vi "CRYCustom Curve Name Replace.vi"(8 "Hardware in":string, 9 "Step Setup in":string, 10 "Setup in":T1={"No.VI"=0, "Category"="", "StepName"="", "Seq setup flattened"="", "Comment"="", "Steps config."=[], "Jump config"=[], "Start"=0.0, "Increment"=0.0, "Name"="Pa", "Unit"="Pa", "Y data"=1, "Y prefix"="", "Y dB ref"=1.0, "Y unit"="", "Repeat State Array"=[]} {"Repeat State Array"."Start" format="%#_5g"; "Y dB ref" format="%.1f"; "Y data" items=["dB", "Lin"]; "Start" format="%#_5g"}, 11 "Type In":string) -> (3 "Inserted Names Out":string[](array[string]))   [LabVIEW 2013]
uses:
  Typedef Control/CRYStep.ctl
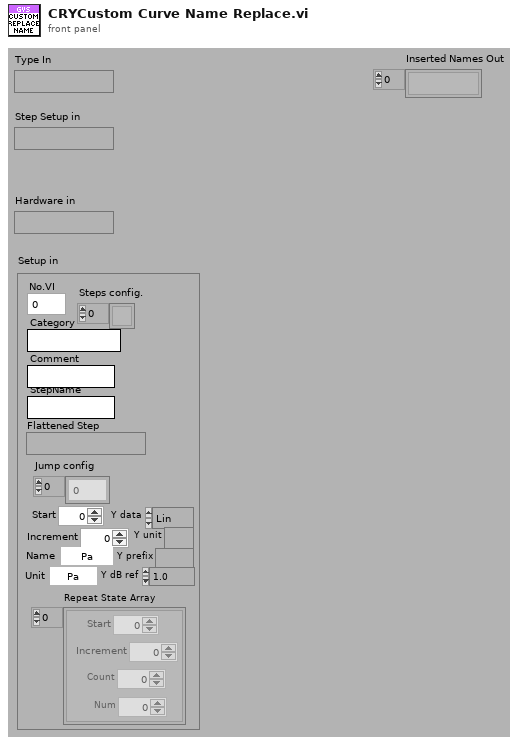
[diagram p1: front panel]
types:
  T1 = typedef "CRYStep.ctl" = cluster{"No.VI":i32, "Category":string, "StepName":string, "Seq setup flattened":string, "Comment":string, "Steps config.":bool[], "Jump config":i32[], "Start":dbl, "Increment":dbl, "Name":string, "Unit":string, "Y data":u16, "Y prefix":string, "Y dB ref":dbl, "Y unit":string, "Repeat State Array":cluster{"Start":dbl, "Increment":dbl, "Count":i32, "Num":i32}[]}
  T2 = cluster{"Type":u16, "Select COM Port":i32, "Byte":i32, "Unit":string, "Curve Name":string}
  T3 = typedef "CRYCustom Cluster.ctl" = cluster{"Help":string, "Flatten Data":string}
  T4 = typedef "CRYData Cluster.ctl" = cluster{"Name":string, "Curve":cluster{"x":dbl, "y":dbl, "z":dbl}[], "X data":u16, "Y data":u16, "Z data":u16, "X axis":u16, "Y axis":u16, "Z axis":u16, "X unit":string, "Y unit":string, "Z unit":string, "X dB ref":dbl, "Y dB ref":dbl, "Z dB ref":dbl, "single val":bool, "protected":bool, "display X":bool, "display Y":bool, "display Z":bool, "Test Info":string, "Step No.":i32, "Plot Settings":cluster{"Color":u32, "Interpolation":u8, "Point Style":u8, "Line Style":u8, "Point Color":u32, "Line Width":u8, "Bar Plot Style":u8, "Fill To":i16}, "AutoProtect":bool}
  T5 = typedef "CRYWaveform Cluster.ctl" = cluster{"Waveform":cluster{"X0":dbl, "dX":dbl, "Y":sgl[]}, "X data":u16, "Y data":u16, "Y axis":u16, "X unit":string, "Y unit":string, "Y dB ref":dbl, "display Y":bool, "display X":bool, "Overload?":bool, "Test Info":string, "Step No.":i32, "Name":string, "protected":bool, "Sqc history":string[], "Signal Channel ID":i32, "Plot Settings":cluster{"Color":u32, "Interpolation":u8, "Point Style":u8, "Line Style":u8, "Point Color":u32, "Line Width":u8, "Bar Plot Style":u8, "Fill To":i16}, "AutoProtect":bool}
  T6 = typedef "CRYResult Cluster.ctl" = cluster{"Name":string, "Margin":dbl, "unit":string, "Verdict":bool, "Limit":string, "Max/Min":string, "protected":bool, "Step No.":i32, "Test Info":string, "AutoProtect":bool}
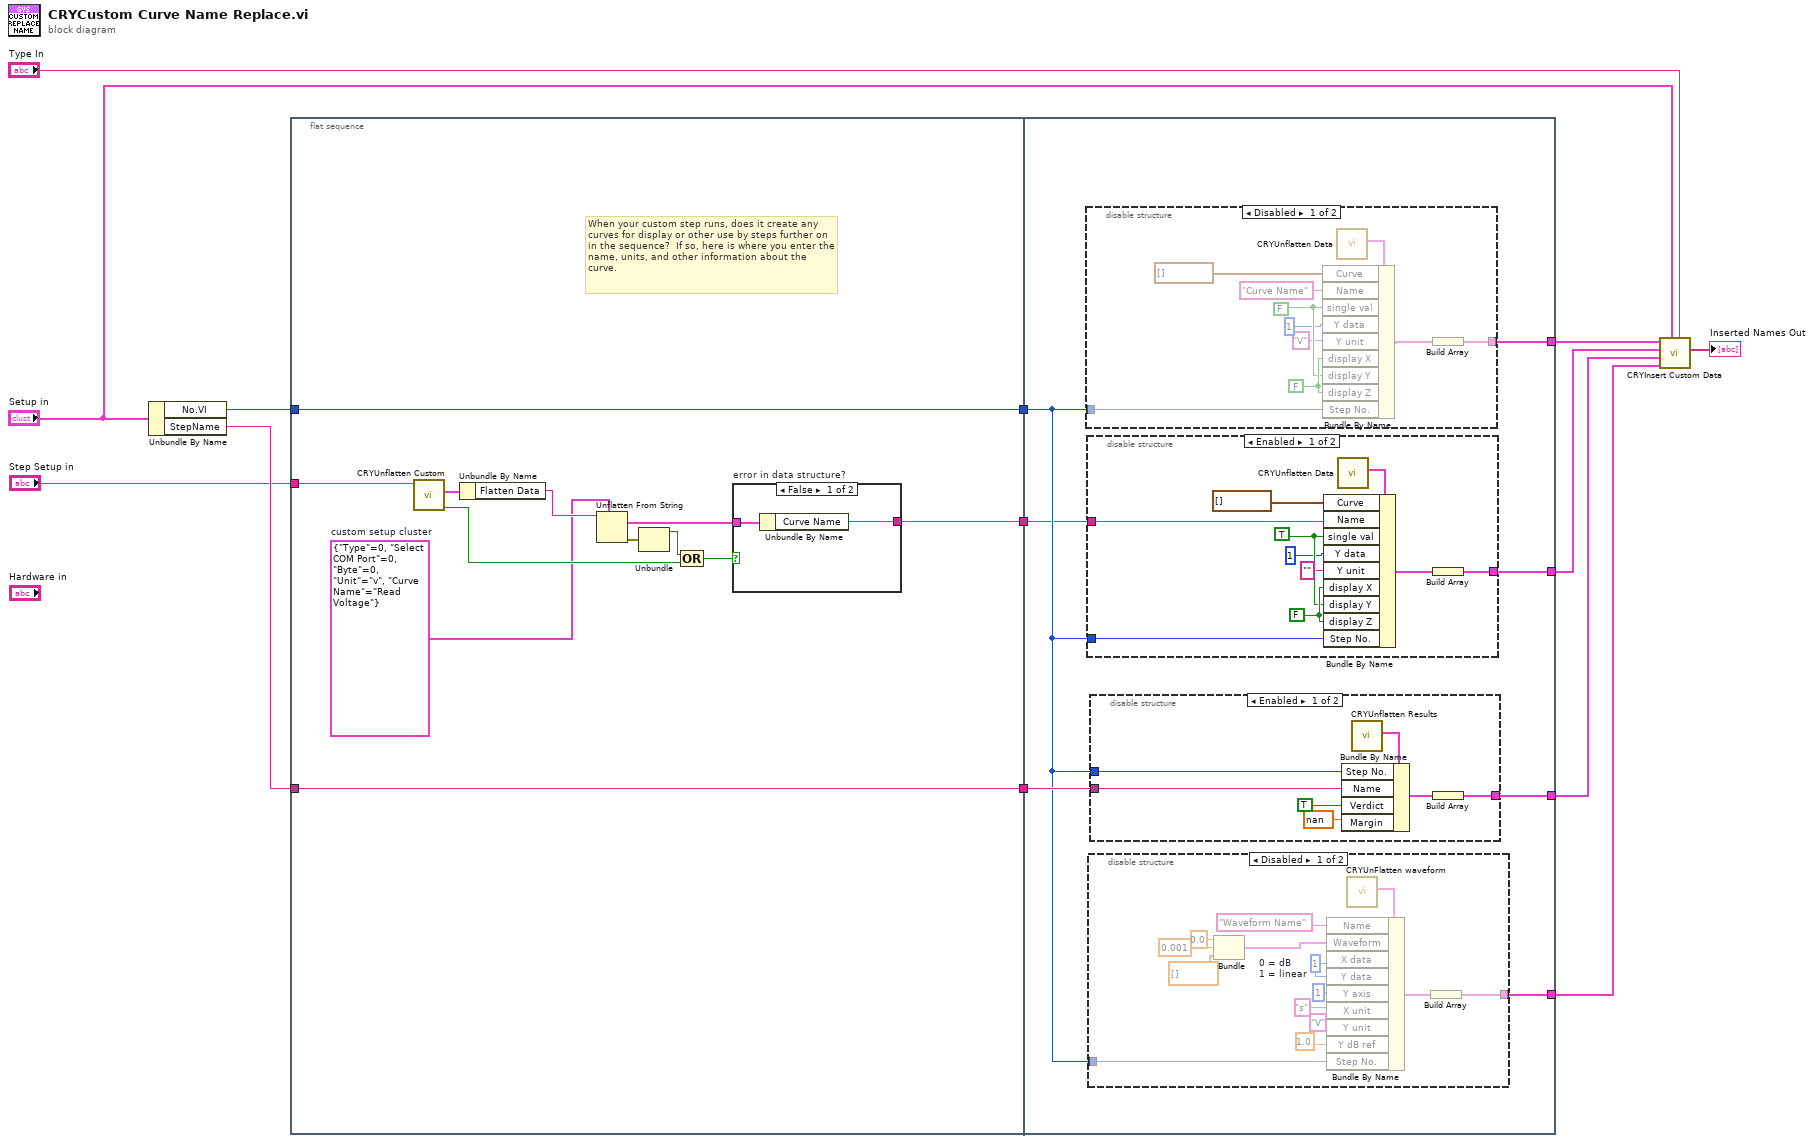
[diagram p0: block diagram]
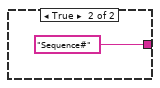
[diagram p2: hidden frame]
diagram:
  n1 = Unbundle By Name("Setup in") -> ("No.VI"=w10:i32, "StepName"=w11:string)
  n2 = flat-sequence {
    tunnel: w10 -> [w24]
    tunnel: w11 -> [w25]
    tunnel: [w25] -> w5
    tunnel: [w24] -> w4
    tunnel: [w19] -> w3
    tunnel: "Step Setup in" -> [w14]
    tunnel: [w33] -> w9
    tunnel: [w32] -> w7
    tunnel: [w31] -> w6
    tunnel: [w30] -> w8
    tunnel: w5 -> [w35]
    tunnel: w4 -> [w34]
    tunnel: w3 -> [w29]
    frame #0 {
      w15 = T2 {"Type"=0, "Select COM Port"=0, "Byte"=0, "Unit"="v", "Curve Name"="Read Voltage"}  # custom setup cluster
      # "When your custom step runs, does it create any curves for display or other use by steps further on in the sequence?  If so, here is where you enter the name, units, and other information about the curve."
      n3 = call "CRYUnflatten Custom.vi"("Unflatten Custom"=w14) -> ("Error?"=w16:bool, "Custom"=w18:T3)  [unwired: 8 in, 1 out]
      n4 = Unbundle By Name(w18) -> ("Flatten Data"=w17:string)
      n5 = Unflatten From String(type=w15, binary string=w17) -> (value=w22:T2, error out=w23:errorcluster)  [unwired: 1 in, 3 out]
      n6 = Unbundle(w23) -> ("status"=w20:bool)  [unwired: 2 out]
      n7 = Compound Arithmetic op=OR(w20, w16) -> (w21:bool)
      n8 = case "error in data structure?" shown="False" w21 {
        tunnel: w22 -> [w27 _]
        tunnel: [w26 "Sequence#" ("Name")] -> w19
        frame False {
          n9 = Unbundle By Name(w27) -> ("Curve Name"=w26:string)
        }
        frame True {
        }
      }
    }
    frame #1 {
      n10 = disable-structure shown="Disabled" {
        disable-tunnel: w34 -> [w41 _]
        disable-tunnel: [w36 _] -> w33
        frame Disabled {
          w44 = FALSE
          w43 = FALSE
          n11 = call "CRYUnflatten Data.vi"() -> ("Datum"=w45:T4)  [unwired: 9 in, 2 out]
          n12 = Bundle By Name(cluster=w45, "Curve"=cluster{"x":dbl, "y":dbl, "z":dbl}[] [] ("appended array"), "Name"="Curve Name", "single val"=w43, "Y data"=u16 1, "Y unit"="V", "display X"=w44, "display Y"=w43, "display Z"=w44, "Step No."=w41) -> (w37:T4)
          n13 = Build Array(w37) -> (w36:T4[])
        }
        frame Enabled {
        }
      }
      n14 = disable-structure shown="Enabled" {
        disable-tunnel: w34 -> [w51 _]
        disable-tunnel: w29 -> [w50 _]
        disable-tunnel: [w48 _] -> w30
        frame Enabled {
          w54 = FALSE
          w53 = TRUE
          n15 = call "CRYUnflatten Data.vi"() -> ("Datum"=w55:T4)  [unwired: 9 in, 2 out]
          n16 = Bundle By Name(cluster=w55, "Curve"=cluster{"x":dbl, "y":dbl, "z":dbl}[] [] ("appended array"), "Name"=w50, "single val"=w53, "Y data"=u16 1, "Y unit"="", "display X"=w54, "display Y"=w53, "display Z"=w54, "Step No."=w51) -> (w49:T4)
          n17 = Build Array(w49) -> (w48:T4[])
        }
        frame Disabled {
        }
      }
      n18 = disable-structure shown="Disabled" {
        disable-tunnel: [w64 _] -> w31
        disable-tunnel: w34 -> [w63 _]
        frame Disabled {
          w69 = u16 1  # 0 = dB 1 = linear
          n19 = Bundle ("Actual waveform data bundle.\nX0\ndX\n[Y] array")(0.0, 0.001, dbl[] []) -> (w73:cluster{dbl, dbl, dbl[]})  [unwired: 1 out]
          n20 = call "CRYUnFlatten waveform.vi"() -> ("Waveform Cluster"=w74:T5)  [unwired: 9 in, 2 out]
          n21 = Bundle By Name(cluster=w74, "Name"="Waveform Name" ("Bundle Element"), "Waveform"=w73, "X data"=w69, "Y data"=w69, "Y axis"=u16 1, "X unit"="s", "Y unit"="V", "Y dB ref"=1.0, "Step No."=w63) -> (w75:T5)
          n22 = Build Array(w75) -> (w64:T5[])
        }
        frame Enabled {
        }
      }
      n23 = disable-structure shown="Enabled" {
        disable-tunnel: w34 -> [w58 _]
        disable-tunnel: w35 -> [w57 _]
        disable-tunnel: [w56 _] -> w32
        frame Enabled {
          n24 = call "CRYUnflatten Results.vi"() -> ("Result"=w59:T6)  [unwired: 9 in, 2 out]
          n25 = Bundle By Name(cluster=w59, "Step No."=w58, "Name"=w57, "Verdict"=TRUE, "Margin"=nan) -> (w61:T6)
          n26 = Build Array(w61) -> (w56:T6[])
        }
        frame Disabled {
        }
      }
    }
  }
  n27 = call "CRYInsert Custom Data.vi"("sAction"="Type In", "Setup in"="Setup in", "Wave"=w6, "Results"=w7, "Values"=w8, "Curves"=w9) -> ("Inserted Names Out"=→"Inserted Names Out":string[])  [unwired: 4 in, 1 out]
